vi "DHE_GetAvailableCmds.vi"(5 "input command":string) -> (6 "remaining":string, 8 "field":string, 10 "parent":string, 12 "SDSU_image_cmds out":string[](array[string]), 13 "SDSU_dhe_cmds out":string[](array[string]), 14 "SDSU_obs_cmds out":string[](array[string]))   [LabVIEW 2016]
panel:
  in  "DHE_obs_cmds":string[](array[string])=["exptime", "display", "fowler", "sur", "coadds", "numreads", "autowrit", "observer", "obstype", "writeframes", "dispframes", "roi", "id", "obsid", "autoobsid", "obsidcounter", "obsidbase", "checkdisk", "chkdisk", "seqdelay", "nsamples", "totdelay", "intdelay", "nightid", "nightidbase", "autonightid", "**ALTERNATIVES**", "displayimage", "display_image", "write_to_disk", "autowrite", "write", "type", "imagestoread", "exposuretime"]
  in  "DHE_dhe_cmds":string[](array[string])=["binning", "readmode", "gainspeed", "artifdata", "config", "state", "timing", "sampling", "autoshutter", "autoclear", "idle", "framesperbuffer", "shutter", "power", "firmware", "controller_info", "readmodes", "samplings", "min_exptime", "read_time", "frame_time", "hard_read_time", "gain", "speed", "artifpattern", "artifpatterns", "link_info", "expvector", "expcode", "bpp", "pixtime", "expasync", "appendid", "arm", "autohandleclear", "deftiming", "**ALTERNATIVES**", "idlemode", "controllerconfig", "timinginfo"]
  in  "DHE_image_cmds":string[](array[string])=["title", "comment", "rootname", "progress", "imnumber", "mext", "geometry", "modifiers", "basename", "directory", "fixed_root", "prefix", "sufix", "id", "expid", "expidbase", "autoid", "autoexpid", "expidcounter", "detext", "tempexptime", "integtime", "**ALTERNATIVES**", "extensions", "multipleextensions", "imagenumber", "imagetitle", "imagecomment", "number", "imageconfig", "tempexptime"]
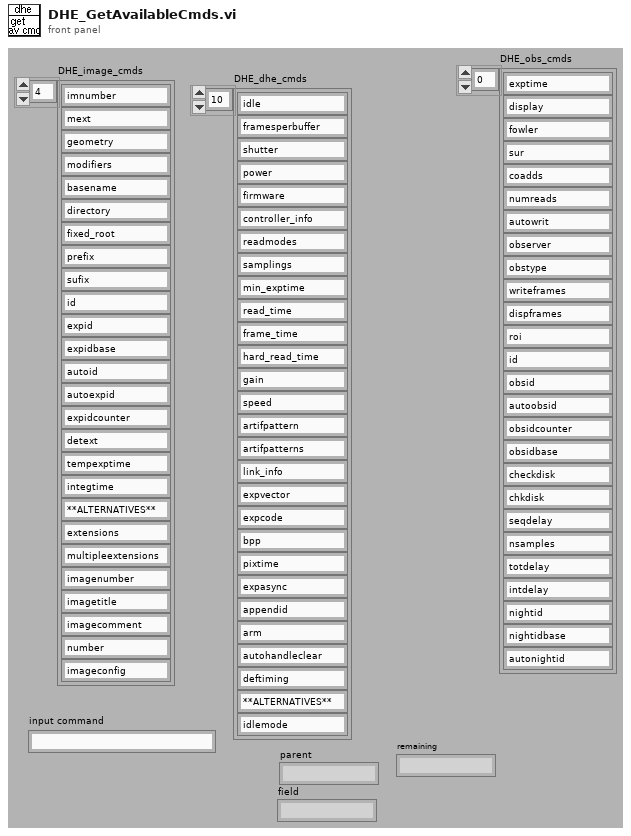
[diagram p1: front panel]
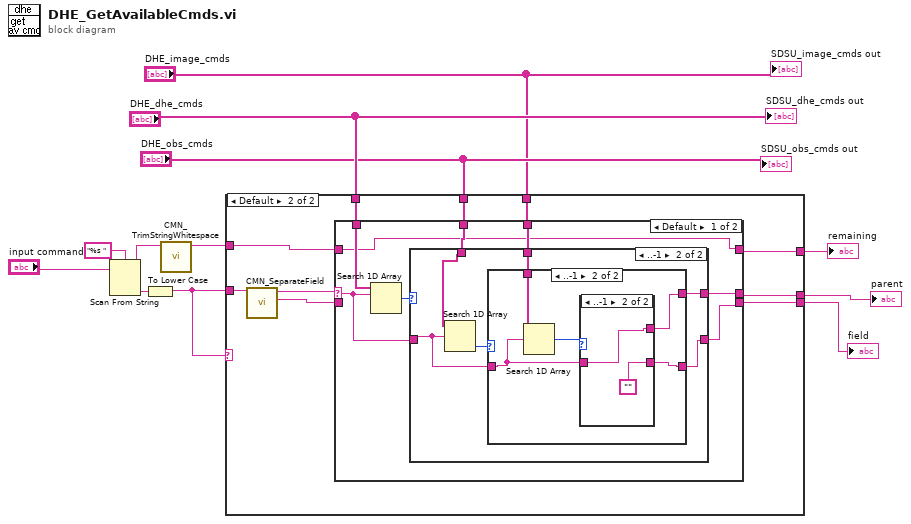
[diagram p0: block diagram]
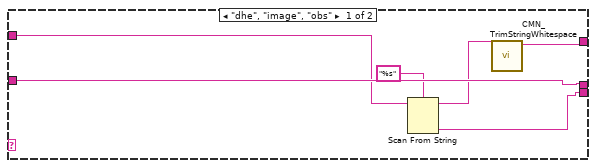
[diagram p2: hidden frame]
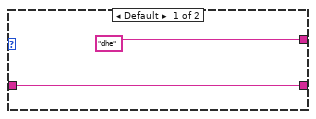
[diagram p3: hidden frame]
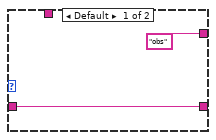
[diagram p4: hidden frame]
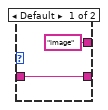
[diagram p5: hidden frame]
diagram:
  n1 = Scan From String(format string="%s " ("Format String"), input string="input command") -> (remaining string=w10:string, output 1=w11:string)  [unwired: 2 in, 3 out]
  n2 = To Lower Case(string=w11) -> (all lower case string=w2:string)
  n3 = call "CMN_TrimStringWhitespace.vi"("string"=w10) -> ("trimmed string"=w7:string)  [unwired: 1 in, 8 out]
  n4 = case shown="Default" w2 {
    tunnel: w2 -> [w18 w28]
    tunnel: "DHE_dhe_cmds" -> [_ w25]
    tunnel: w7 -> [w17 w24]
    tunnel: [w13 w23] -> w6
    tunnel: [w18 w22] -> w5
    tunnel: [w15 w21] -> w4
    tunnel: "DHE_obs_cmds" -> [_ w20]
    tunnel: "DHE_image_cmds" -> [_ w19]
    frame "dhe", "image", "obs" {
      n5 = Scan From String(format string="%s", input string=w17) -> (remaining string=w14:string, output 1=w15:string)  [unwired: 2 in, 3 out]
      n6 = call "CMN_TrimStringWhitespace.vi"("string"=w14) -> ("trimmed string"=w13:string)  [unwired: 1 in, 8 out]
    }
    frame Default {
      n7 = call "CMN_SeparateField.vi"("input arg"=w28) -> ("field"=w26:string, "parent"=w27:string)  [unwired: 3 in, 6 out]
      n8 = case shown="Default" w27 {
        selector: w27 -> [w33 w58]
        tunnel: w26 -> [_ w57]
        tunnel: w25 -> [w36 _]
        tunnel: [w34 w58] -> w22
        tunnel: [w32 w57] -> w21
        tunnel: [w29 w56] -> w23
        tunnel: w24 -> [w29 w56]
        tunnel: w20 -> [w31 _]
        tunnel: w19 -> [w30 _]
        frame Default {
          n9 = Search 1D Array(1D array=w36, element=w33) -> (index of element=w35:i32)  [unwired: 1 out]
          n10 = case shown="..-1" w35 {
            tunnel: ["dhe" w41] -> w34
            tunnel: w33 -> [w37 w40]
            tunnel: [w37 w39] -> w32
            tunnel: w31 -> [_ w44]
            tunnel: w30 -> [_ w42]
            frame Default {
            }
            frame ..-1 {
              n11 = Search 1D Array(1D array=w44, element=w40) -> (index of element=w43:i32)  [unwired: 1 out]
              n12 = case shown="..-1" w43 {
                tunnel: w42 -> [_ w51]
                tunnel: ["obs" w49] -> w41
                tunnel: w40 -> [w45 w48]
                tunnel: [w45 w47] -> w39
                frame Default {
                }
                frame ..-1 {
                  n13 = Search 1D Array(1D array=w51, element=w48) -> (index of element=w50:i32)  [unwired: 1 out]
                  n14 = case shown="..-1" w50 {
                    tunnel: ["image" w55] -> w49
                    tunnel: [w52 ""] -> w47
                    tunnel: w48 -> [w52 w55]
                    frame Default {
                    }
                    frame ..-1 {
                    }
                  }
                }
              }
            }
          }
        }
        frame "dhe", "image", "obs" {
        }
      }
    }
  }
  "remaining" <- w6
  "parent" <- w5
  "field" <- w4
  "SDSU_image_cmds out" <- "DHE_image_cmds"
  "SDSU_dhe_cmds out" <- "DHE_dhe_cmds"
  "SDSU_obs_cmds out" <- "DHE_obs_cmds"
